vi "fakeLineCreation.vi"(8 "volume info":T2, 9 "data stream in":u32[](array[numeric]), 11 "voxel number":u32) -> (0 "line":T1, 1 "data stream out":u32[](array[numeric]), 3 "voxel number out":u32)   [LabVIEW 2010]
uses:
  line_info.ctl
panel:
  out "zi":u32
  out "xi":u32
  out "yi":u32
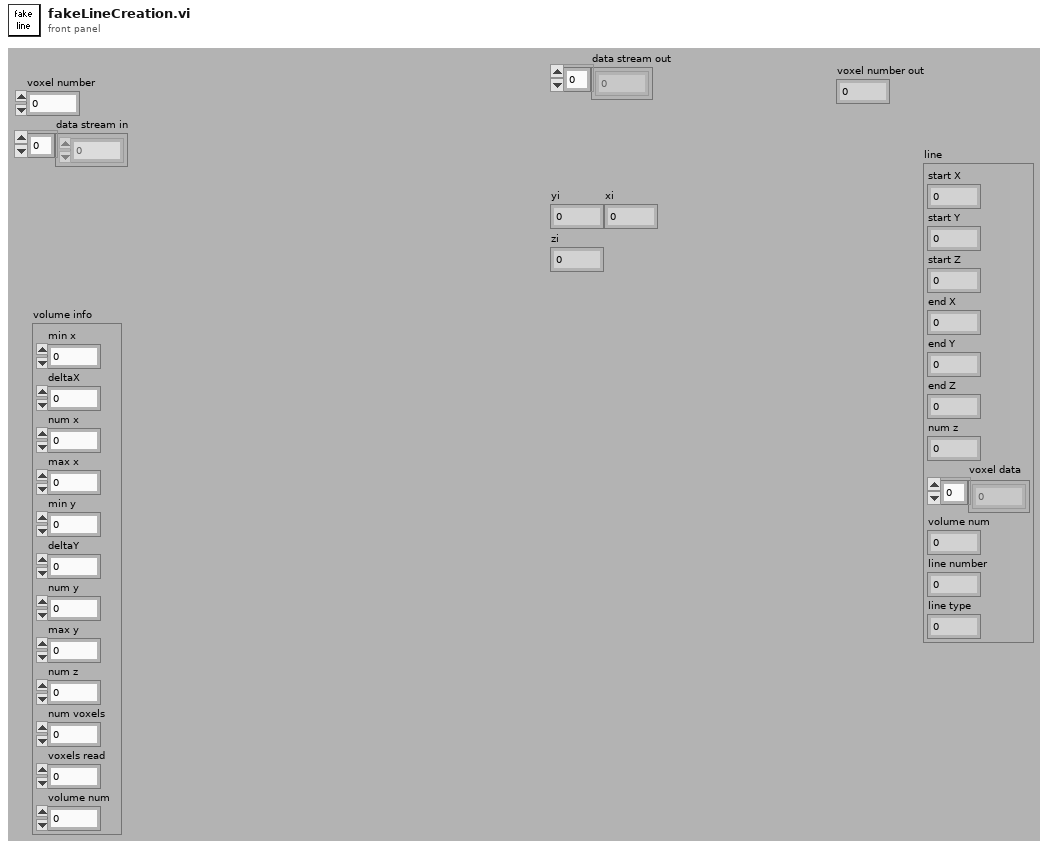
[diagram p1: front panel]
types:
  T1 = typedef "line_info.ctl" = cluster{"start X":i16, "start Y":i16, "start Z":i16, "end X":i16, "end Y":i16, "end Z":i16, "num z":u8, "voxel data":u32[], "volume num":u32, "line number":u16, "line type":u16}
  T2 = cluster{"min x":i16, "deltaX":dbl, "num x":u32, "max x":i16, "min y":i16, "deltaY":dbl, "num y":u32, "max y":i16, "num z":u32, "num voxels":u32, "voxels read":u32, "volume num":u32}
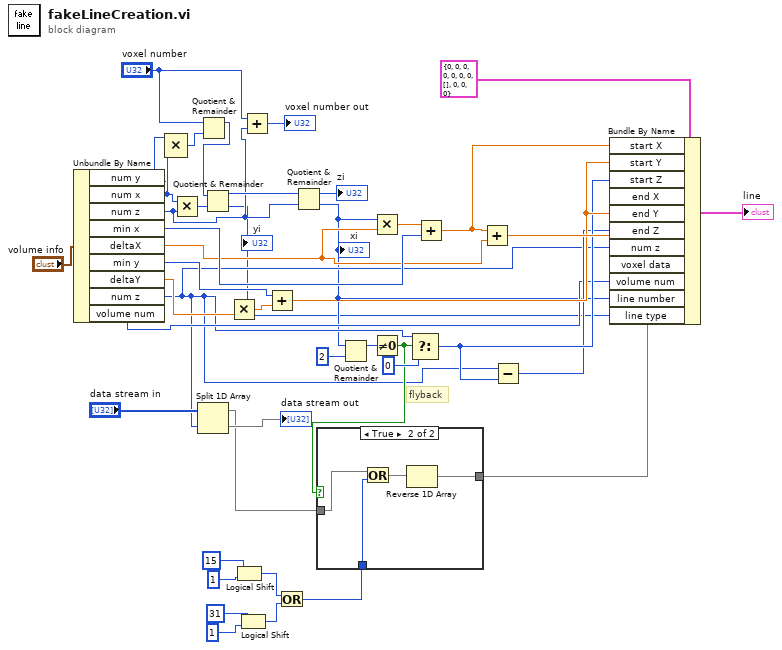
[diagram p0: block diagram]
diagram:
  # "flyback"
  n1 = Unbundle By Name("volume info") -> ("num y"=w16:u32, "num x"=w15:u32, "num z"=w14:u32, "min x"=w37:i16, "deltaX"=w35:dbl, "min y"=w31:i16, "deltaY"=w33:dbl, "num z"=w3:u32, "volume num"=w7:u32)
  n2 = Compound Arithmetic op=MULTIPLY(w16, w15, w14) -> (w12:u32)
  n3 = Multiply(x=w15, y=w14) -> (x*y=w41:u32)
  n4 = Split 1D Array(array="data stream in", index=w3) -> (first subarray=w4:u32[], second subarray=→"data stream out":u32[])
  n5 = Quotient & Remainder(x="voxel number", y=w12) -> (x-y*floor(x/y)=w13:u32)  [unwired: 1 out]
  n6 = Quotient & Remainder(x=w13, y=w41) -> (x-y*floor(x/y)=w40:u32, floor(x/y)=w1:u32)
  "yi" <- w1
  n7 = Multiply(x=w1, y=w33) -> (x*y=w32:dbl)
  n8 = Logical Shift(y=i8 15, x=u32 1) -> (x << y=w20:u32)
  n9 = Logical Shift(y=i8 31, x=u32 1) -> (x << y=w19:u32)
  n10 = Add(x="voxel number", y=w14) -> (x+y=→"voxel number out":u32)
  n11 = Add(x=w31, y=w32) -> (x+y=w30:dbl)
  n12 = Or(x=w20, y=w19) -> (x .or. y?=w10:u32)
  n13 = Quotient & Remainder(x=w40, y=w14) -> (x-y*floor(x/y)=→"zi":u32, floor(x/y)=w2:u32)
  "xi" <- w2
  n14 = Quotient & Remainder(x=w2, y=u32 2) -> (x-y*floor(x/y)=w28:u32)  [unwired: 1 out]
  n15 = Multiply(x=w2, y=w35) -> (x*y=w38:dbl)
  n16 = Not Equal To 0?(x=w28) -> (x != 0?=w11:bool)
  n17 = case shown="True" w11 {
    tunnel: w4 -> [w44 w48]
    tunnel: w10 -> [_ w47]
    tunnel: [w44 w45] -> w9
    frame False {
    }
    frame True {
      n18 = Or(x=w48, y=w47) -> (x .or. y?=w46:u32[])
      n19 = Reverse 1D Array(array=w46) -> (reversed array=w45:u32[])
    }
  }
  n20 = Select(t=w3, s=w11, f=u32 0) -> (s? t:f=w26:u32)
  n21 = Add(x=w38, y=w37) -> (x+y=w36:dbl)
  n22 = Add(x=w36, y=w35) -> (x+y=w34:dbl)
  n23 = Subtract(x=w3, y=w26) -> (x-y=w25:u32)
  n24 = Bundle By Name(cluster=T1 {"start X"=0, "start Y"=0, "start Z"=0, "end X"=0, "end Y"=0, "end Z"=0, "num z"=0, "voxel data"=[], "volume num"=0, "line number"=0, "line type"=0} ("line"), "start X"=w36, "start Y"=w30, "start Z"=w26, "end X"=w34, "end Y"=w30, "end Z"=w25, "num z"=w3, "voxel data"=w9, "volume num"=w7, "line number"=w2, "line type"=w1) -> (→"line":T1)
